vi "Analysis Results.vi"(6 "Image Nr.":i32, 8 "error in (no error)":errorcluster, 9 "Results In":refnum<class "Analyze Results Base.lvclass">[](array[class]), 10 "Parameters":refnum<class "Analyze Parameter Base.lvclass">[](array[class]), 11 "HIJ Vision Camera App In":refnum<class "HIJ Vision Camera App.lvclass">) -> (0 "error out":errorcluster, 3 "HIJ Vision Camera App Out":refnum<class "HIJ Vision Camera App.lvclass">)   [LabVIEW 2020, in "HIJ Vision Camera App.lvlib" / "HIJ Vision Camera App.lvclass"]
uses:
  HIJ Vision Camera App.lvclass
  C:/Users/AlexK/work/LabVIEW Programme/POLARIS CAM Log Abw und E/Submodules/HIJ Vision/Application Base Actors/HIJ Vision Application/HIJ Vision Application/HIJ Vision Application.lvclass
  C:/Program Files (x86)/National Instruments/LabVIEW 2020/vi.lib/ActorFramework/Actor/Actor.lvclass
  Analyze/Results and Overlays/Results Base/Analyze Results Base.lvclass
  Analyze/Analyze Parameter/Analyze Parameter Base/Analyze Parameter Base.lvclass
  HIJ Vision Camera App Dialog/HIJ Vision Camera App Dialog Messages/Sequence State Msg/Sequence State Msg.lvclass
  C:/Users/AlexK/work/LabVIEW Programme/POLARIS CAM Log Abw und E/Submodules/HIJ Vision/Application Base Actors/HIJ Vision Camera App/HIJ Vision Camera App Messages/Sequence State Msg/Sequence State Msg.lvclass
  HIJ Vision Application/HIJ Vision Application/HIJ Vision Application.lvclass/HIJ Vision Application.ctl
  <vilib>/ActorFramework/Actor/Actor.lvclass/Actor.ctl
  HIJ Vision Camera App.lvclass/HIJ Vision Camera App.ctl
  <vilib>/ActorFramework/Message Enqueuer/Message Enqueuer.lvclass/Message Enqueuer.ctl
  HIJ Vision Camera App Messages/Sequence State Msg/Sequence State Msg.lvclass/Sequence State Msg.ctl
  HIJ Vision Application/HIJ Vision Application/Read Display Enq.vi
  <vilib>/ActorFramework/Message Enqueuer/Enqueue.vi
  Display Actors/HIJ Vision Display/HIJ Vision Display Messages/Save Image Msg/Save Image Msg.lvclass
  C:/Program Files (x86)/National Instruments/LabVIEW 2020/vi.lib/ActorFramework/Message/Message.lvclass
  HIJ Vision Camera App Messages/Sequence State Msg/Sequence State Msg.lvclass
  <vilib>/ActorFramework/Message Priority Queue/Priority Enqueue.vi
  HIJ Vision Application/HIJ Vision Application/HIJ Vision Application.lvclass
  <vilib>/ActorFramework/Message Enqueuer/Message Enqueuer.lvclass
  <vilib>/ActorFramework/Actor/Actor.lvclass
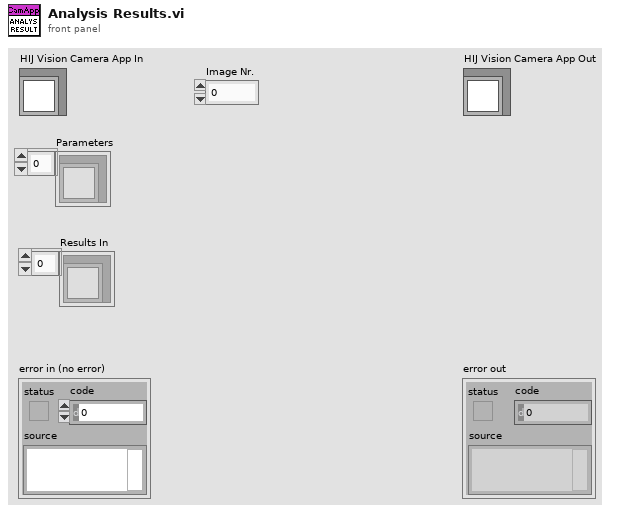
[diagram p1: front panel]
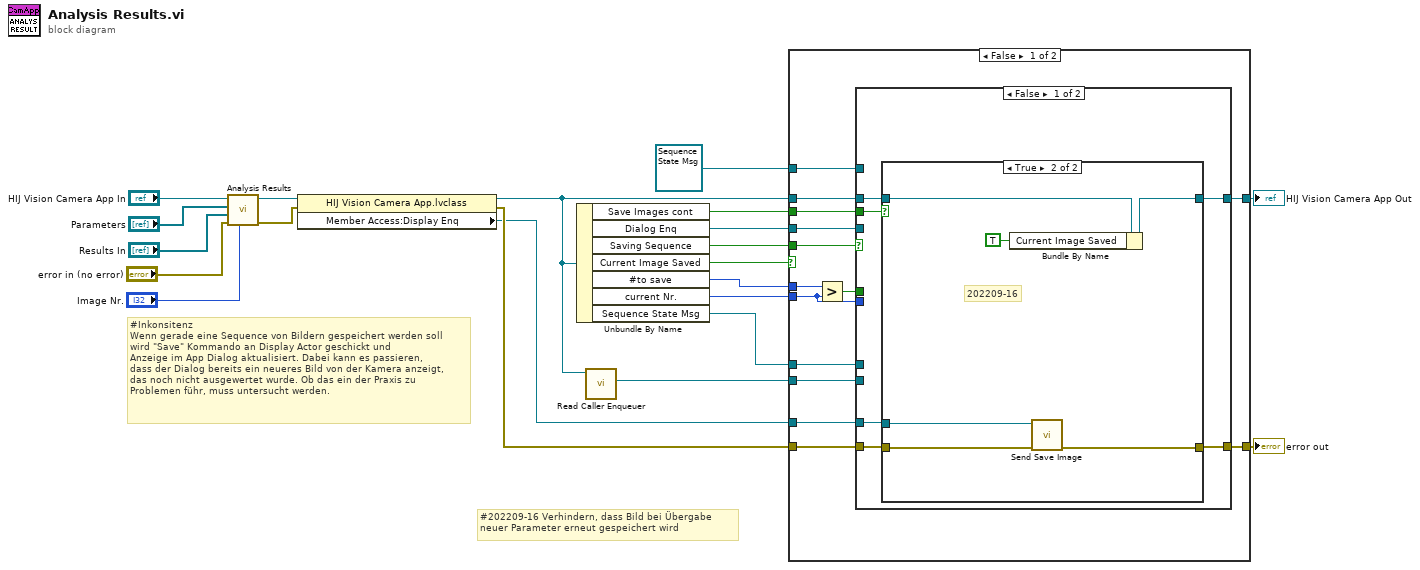
[diagram p0: block diagram]
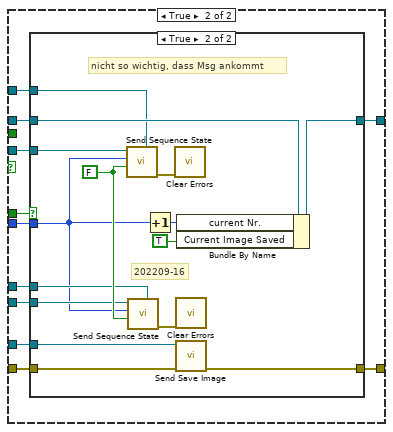
[diagram p3: hidden frame]
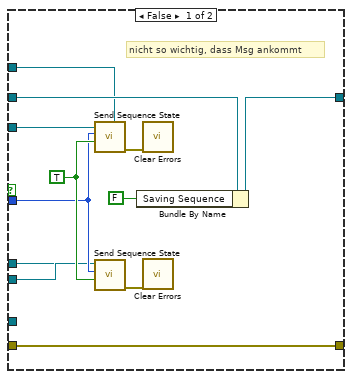
[diagram p4: hidden frame]
diagram:
  # "#202209-16 Verhindern, dass Bild bei Übergabe \nneuer Parameter erneut gespeichert wird"
  # "#Inkonsitenz \nWenn gerade eine Sequence von Bildern gespeichert werden soll\nwird \"Save\" Kommando an Display Actor geschickt und\nAnzeige im App Dialog aktualisiert. Dabei kann es passieren,\ndass der Dialog bereits ein neueres Bild von der Kamera anzeigt,\ndas noch nicht ausgewertet wurde. Ob das ein der Praxis zu \nProblemen führ, muss untersucht werden."
  n1 = call-parent "Analysis Results.vi"("Image Nr."="Image Nr.", "error in (no error)"="error in (no error)", "Results In"="Results In", "Parameters"="Parameters", "Launch IMAQ Display in"="HIJ Vision Camera App In") -> ("error out"=w1:errorcluster, "Launch IMAQ Display out"=w6:refnum<class "HIJ Vision Camera App.lvclass">)  [unwired: 5 in]
  n2 = property class="HIJ Vision Camera App.lvclass"(reference=w6, error in=w1) -> (reference out=w9:refnum<class "HIJ Vision Camera App.lvclass">, error out=w21:errorcluster, "Member Access:Display Enq"=w17:refnum<class "Message Enqueuer.lvclass">)
  n3 = Unbundle By Name(w9) -> ("Save Images cont"=w12:bool, "Dialog Enq"=w13:refnum<class "Message Enqueuer.lvclass">, "Saving Sequence"=w19:bool, "Current Image Saved"=w7:bool, "#to save"=w18:i32, "current Nr."=w14:i32, "Sequence State Msg"=w10:refnum<class "Sequence State Msg.lvclass">)
  n4 = call <vilib>:"Read Caller Enqueuer.vi"("Actor"=w9) -> ("Caller Enqueuer"=w8:refnum<class "Message Enqueuer.lvclass">)  [unwired: 10 in]
  n5 = case shown="False" w7 {
    tunnel: w21 -> [w35 w88]
    tunnel: w19 -> [w34 _]
    tunnel: w18 -> [w33 _]
    tunnel: w17 -> [w31 _]
    tunnel: [w30 w88] -> w16
    tunnel: [w29 w89] -> w15
    tunnel: w14 -> [w28 _]
    tunnel: w13 -> [w27 _]
    tunnel: w12 -> [w26 _]
    tunnel: refnum<class "Sequence State Msg.lvclass"> refnum ("HIJ Vision Camera App Dialog.lvlib:Sequence State Msg.lvclass") -> [w25 _]
    tunnel: w10 -> [w24 _]
    tunnel: w9 -> [w23 w89]
    tunnel: w8 -> [w22 _]
    frame False {
      n6 = Greater?(x=w33, y=w28) -> (0:w32:bool)
      n7 = case shown="False" w34 {
        tunnel: w32 -> [_ w60]
        tunnel: w31 -> [w36 w59]
        tunnel: w35 -> [w37 w58]
        tunnel: [w38 w57] -> w30
        tunnel: w23 -> [w39 w56]
        tunnel: [w40 w55] -> w29
        tunnel: w28 -> [_ w54]
        tunnel: w27 -> [_ w53]
        tunnel: w26 -> [w41 _]
        tunnel: w25 -> [_ w52]
        tunnel: w24 -> [_ w51]
        tunnel: w22 -> [_ w50]
        frame False {
          n8 = case shown="True" w41 {
            tunnel: [w43 w45] -> w40
            tunnel: w39 -> [w43 w49]
            tunnel: [w42 w47] -> w38
            tunnel: w37 -> [w42 w48]
            tunnel: w36 -> [_ w46]
            frame False {
            }
            frame True {
              # "202209-16"
              n9 = Bundle By Name(cluster=w49, "Current Image Saved"=TRUE) -> (w45:refnum<class "HIJ Vision Camera App.lvclass">)
              n10 = call "Send Save Image.vi"("error in (no error)"=w48, "Message Enqueuer"=w46) -> ("error out"=w47:errorcluster)  [unwired: 8 in, 1 out]
            }
          }
        }
        frame True {
          n11 = case shown="True" w60 {
            tunnel: w59 -> [_ w85]
            tunnel: w58 -> [w70 w84]
            tunnel: [w70 w83] -> w57
            tunnel: w56 -> [w67 w82]
            tunnel: [w69 w81] -> w55
            tunnel: w54 -> [w71 w74]
            tunnel: w53 -> [w65 w86]
            tunnel: w52 -> [w64 w78]
            tunnel: w51 -> [w61 w76]
            tunnel: w50 -> [w62 w77]
            frame False {
              w72 = TRUE ("Ready?")
              # "nicht so wichtig, dass Msg ankommt"
              n12 = call "Send Sequence State.vi"("Msg Type"=w64, "Ready?"=w72, "Current Nr."=w71, "Message Enqueuer"=w65) -> ("error out"=w66:errorcluster)  [unwired: 6 in, 1 out]
              n13 = call "Send Sequence State.vi"("Msg Type"=w61, "Ready?"=w72, "Current Nr."=w71, "Message Enqueuer"=w62) -> ("error out"=w63:errorcluster)  [unwired: 6 in, 1 out]
              n14 = Bundle By Name(cluster=w67, "Saving Sequence"=FALSE) -> (w69:refnum<class "HIJ Vision Camera App.lvclass">)
              n15 = call <vilib>:"Clear Errors.vi"("error in (no error)"=w66) -> ()  [unwired: 5 in, 2 out]
              n16 = call <vilib>:"Clear Errors.vi"("error in (no error)"=w63) -> ()  [unwired: 5 in, 2 out]
            }
            frame True {
              w87 = FALSE ("Ready?")
              # "202209-16"
              # "nicht so wichtig, dass Msg ankommt"
              n17 = call "Send Sequence State.vi"("Msg Type"=w78, "Ready?"=w87, "Current Nr."=w74, "Message Enqueuer"=w86) -> ("error out"=w79:errorcluster)  [unwired: 6 in, 1 out]
              n18 = call "Send Sequence State.vi"("Msg Type"=w76, "Ready?"=w87, "Current Nr."=w74, "Message Enqueuer"=w77) -> ("error out"=w75:errorcluster)  [unwired: 6 in, 1 out]
              n19 = Increment(x=w74) -> (x+1=w80:i32)
              n20 = call <vilib>:"Clear Errors.vi"("error in (no error)"=w79) -> ()  [unwired: 5 in, 2 out]
              n21 = call <vilib>:"Clear Errors.vi"("error in (no error)"=w75) -> ()  [unwired: 5 in, 2 out]
              n22 = call "Send Save Image.vi"("error in (no error)"=w84, "Message Enqueuer"=w85) -> ("error out"=w83:errorcluster)  [unwired: 8 in, 1 out]
              n23 = Bundle By Name(cluster=w82, "current Nr."=w80, "Current Image Saved"=TRUE) -> (w81:refnum<class "HIJ Vision Camera App.lvclass">)
            }
          }
        }
      }
    }
    frame True {
    }
  }
  "error out" <- w16
  "HIJ Vision Camera App Out" <- w15
